vi "getMagnetVector.vi"(8 "error in (no error)":errorcluster, 11 "Instrument.Cryostat in":refnum<class "Instrument.Cryostat.lvclass">) -> (0 "error out":errorcluster, 1 "Status":string, 2 "Field (T)":dbl[](array[numeric]), 3 "Instrument.Cryostat out":refnum<class "Instrument.Cryostat.lvclass">, 4 "Finished?":bool)   [LabVIEW 2019, in "Instrument.Cryostat.lvclass"]
uses:
  Instrument.Cryostat.lvclass
  Instrument/Instrument.lvclass
  d99fca9a-0ec4-4724-b19e-b90548b9cfa0.vi
  Typedefs/getMagnetVector--cluster.ctl
  C:/Users/patrick/Documents/GitHub/Instrument-Framework/lvsrc/Instrument/Instrument.lvclass
  C:/Program Files (x86)/National Instruments/LabVIEW 2019/vi.lib/JKI/JKI SMO/SMO/SMO.lvclass
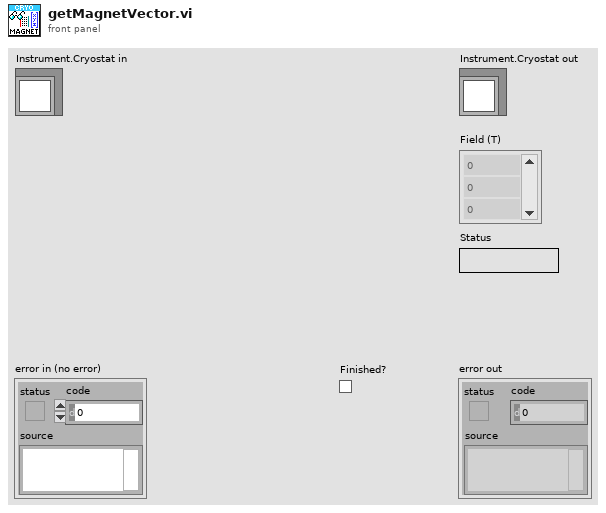
[diagram p1: front panel]
types:
  T1 = typedef "Instrument.Cryostat.lvclass/getMagnetVector--cluster.ctl" = cluster{"Field (T)":dbl[], "Status":string, "Finished?":bool}
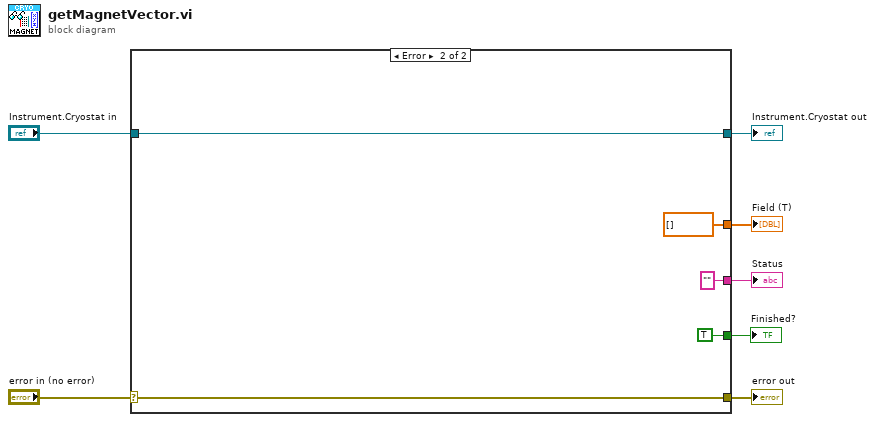
[diagram p0: block diagram]
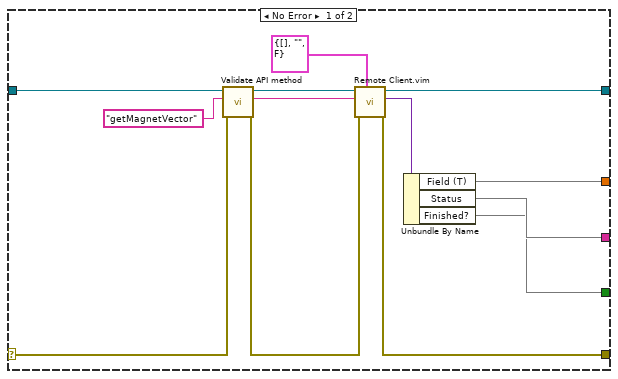
[diagram p2: hidden frame]
diagram:
  n1 = case shown="Error" "error in (no error)" {
    selector: "error in (no error)" -> [w16 w25]
    tunnel: [w14 w25] -> w6
    tunnel: [w13 w24] -> w4
    tunnel: "Instrument.Cryostat in" -> [w17 w24]
    tunnel: [w11 dbl[] [] ("Field (T)")] -> w3
    tunnel: [w10 "" ("Status")] -> w2
    tunnel: [w9 TRUE] -> w1
    frame No Error {
      n2 = call "Validate API method.vi"("error in (no error)"=w16, "command in"="getMagnetVector" ("error message (\"\")"), "Instrument in"=w17) -> ("error out"=w15:errorcluster, "command out"=w19:string, "Instrument out"=w18:refnum<class "Instrument.Cryostat.lvclass">)  [unwired: 6 in]
      n3 = call "Remote Client.vim"("Data Out type"=T1 {"Field (T)"=[], "Status"="", "Finished?"=FALSE} ("getMagnet"), "error in (no error)"=w15, "method"=w19, "Instrument in"=w18) -> ("error out"=w14:errorcluster, "Data out"=w12:variant, "Instrument out"=w13:refnum<class "Instrument.Cryostat.lvclass">)  [unwired: 4 in, 1 out]
      n4 = Unbundle By Name(w12) -> ("Field (T)"=w11, "Status"=w10, "Finished?"=w9)
    }
    frame Error {
    }
  }
  "error out" <- w6
  "Instrument.Cryostat out" <- w4
  "Field (T)" <- w3
  "Status" <- w2
  "Finished?" <- w1
